vi "ELOG_Channels_Get.vi"(8 "error in (no error)":errorcluster, 11 "OXY_SCPI Reseource In":refnum<visa-resource-name>) -> (0 "error out":errorcluster, 1 "communication_data":T1, 2 "Channel Item List":string[](array[string]), 3 "OXY_SCPI Reseource Out":refnum<visa-resource-name>)   [LabVIEW 2018, in "OXYGEN.lvlib"]
doc: "Returns the current list of requested channels."
uses:
  OXYGEN.lvlib
  TypeDefs/Cluster_RawCommData.ctl
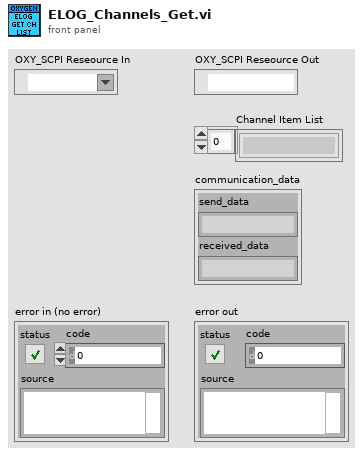
[diagram p1: front panel]
types:
  T1 = typedef "OXYGEN.lvlib/Cluster_RawCommData.ctl" = cluster{"send_data":string, "received_data":string}
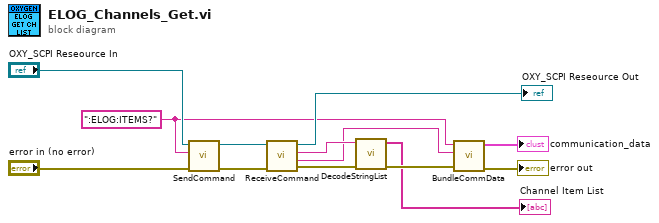
[diagram p0: block diagram]
diagram:
  w1 = ":ELOG:ITEMS?" ("String to Send")
  n1 = call "SendCommand.vi"("error in (no error)"="error in (no error)", "String to Send"=w1, "OXY_SCPI Reseource In"="OXY_SCPI Reseource In") -> ("error out"=w13:errorcluster, "OXY_SCPI Reseource Out"=w12:refnum<visa-resource-name>)  [unwired: 7 in]
  n2 = call "ReceiveCommand.vi"("error in (no error)"=w13, "OXY_SCPI Reseource In"=w12) -> ("error out"=w6:errorcluster, "received Data with Header"=w2:string, "received Data"=w5:string, "OXY_SCPI Reseource Out"=→"OXY_SCPI Reseource Out":refnum<visa-resource-name>)  [unwired: 6 in]
  n3 = call "DecodeStringList.vi"("error in (no error)"=w6, "String List (\"<STR1>\",\"<STR2>\",...)"=w5) -> ("error out"=w4:errorcluster, "String as Array"=→"Channel Item List":string[])  [unwired: 8 in]
  n4 = call "BundleCommData.vi"("error in (no error)"=w4, "received_data"=w2, "send_data"=w1) -> ("error out"=→"error out":errorcluster, "communication_data"=→"communication_data":T1)  [unwired: 7 in]
